vi "ALS control local.vi"(0 "DDE control":i8, 1 "ChemStation Name":string="hpcore7544", 2 "ALS method folder":path=path "C:/Chem32/1/METHODS/YM_SAMPLEPREP.M") -> ()   [LabVIEW 2017]
panel:
  # "Only use this VI on the PC where ChemStation is installed."
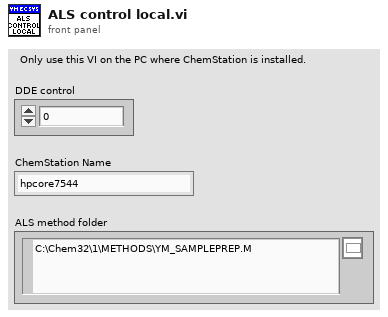
[diagram p1: front panel]
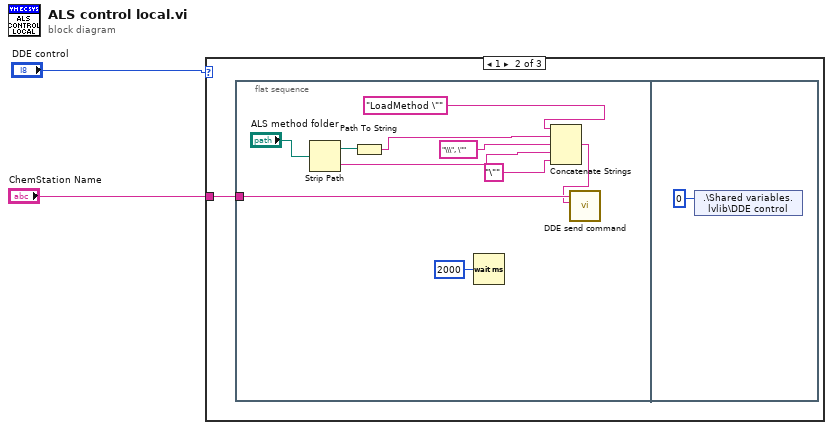
[diagram p0: block diagram]
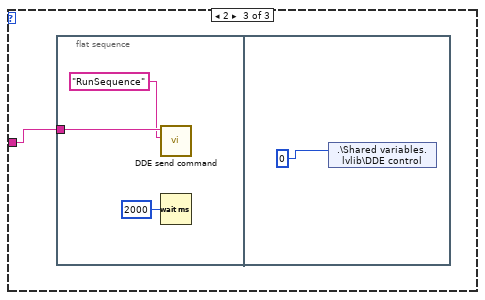
[diagram p3: hidden frame]
diagram:
  n1 = case shown="1" "DDE control" {
    tunnel: "ChemStation Name" -> [_ w3 w15]
    frame 0, Default {
    }
    frame 1 {
      n2 = flat-sequence {
        tunnel: w3 -> [w12]
        frame #0 {
          n3 = Strip Path(path="ALS method folder") -> (stripped path=w8:path, name=w5:string)
          n4 = Path To String(path=w8) -> (string=w7:string)
          n5 = Wait (ms)(milliseconds to wait=u32 2000) -> ()  [unwired: 1 out]
          n6 = Concatenate Strings("LoadMethod \"", w7, "\\\", \"" ("string"), w5, "\"" ("string")) -> (w11:string)
          n7 = call "DDE send command.vi"("Command"=w11, "ChemStation Name"=w12) -> ()  [unwired: 10 in]
        }
        frame #1 {
          n8 = shared-variable ".\\Shared variables.lvlib\\DDE control"(i8 0 ("DDE control")) -> ()  [unwired: 1 in, 1 out]
        }
      }
    }
    frame 2 {
      n9 = flat-sequence {
        tunnel: w15 -> [w18]
        frame #0 {
          n10 = call "DDE send command.vi"("Command"="RunSequence", "ChemStation Name"=w18) -> ()  [unwired: 10 in]
          n11 = Wait (ms)(milliseconds to wait=u32 2000) -> ()  [unwired: 1 out]
        }
        frame #1 {
          n12 = shared-variable ".\\Shared variables.lvlib\\DDE control"(i8 0 ("data in")) -> ()  [unwired: 1 in, 1 out]
        }
      }
    }
  }
